vi "BuildPlotsOneGraph.vi"(0 "PlotCommand":string, 1 "Desired Legends":string[](array[string]), 2 "Error Bar Type":T1, 5 "Plotstyles":T3[](array[typedef]) {"LineType" min=1 max=6 step=1; "LineWidth" min=1 max=6 step=1; "PointSize" min=0 step=0.1}, 7 "PlotNamesNeed $$?":bool=TRUE, 9 "Plot Legends":string[](array[string]), 11 "PlotArray":cluster{dbl[], dbl[]}[](array[cluster]), 12 "Legend":string[](array[string]), 13 "Error Bar Cluster":T2[](array[typedef])) -> (4 "String out":string, 6 "Xspan":cluster{"Max":dbl, "Min":dbl}, 10 "Yspan":cluster{"Max":dbl, "Min":dbl})   [LabVIEW 2016]
uses:
  plotstyle.ctl
  Error_bars.ctl
  Error bar Type.ctl
  Results_plotter_Global.vi
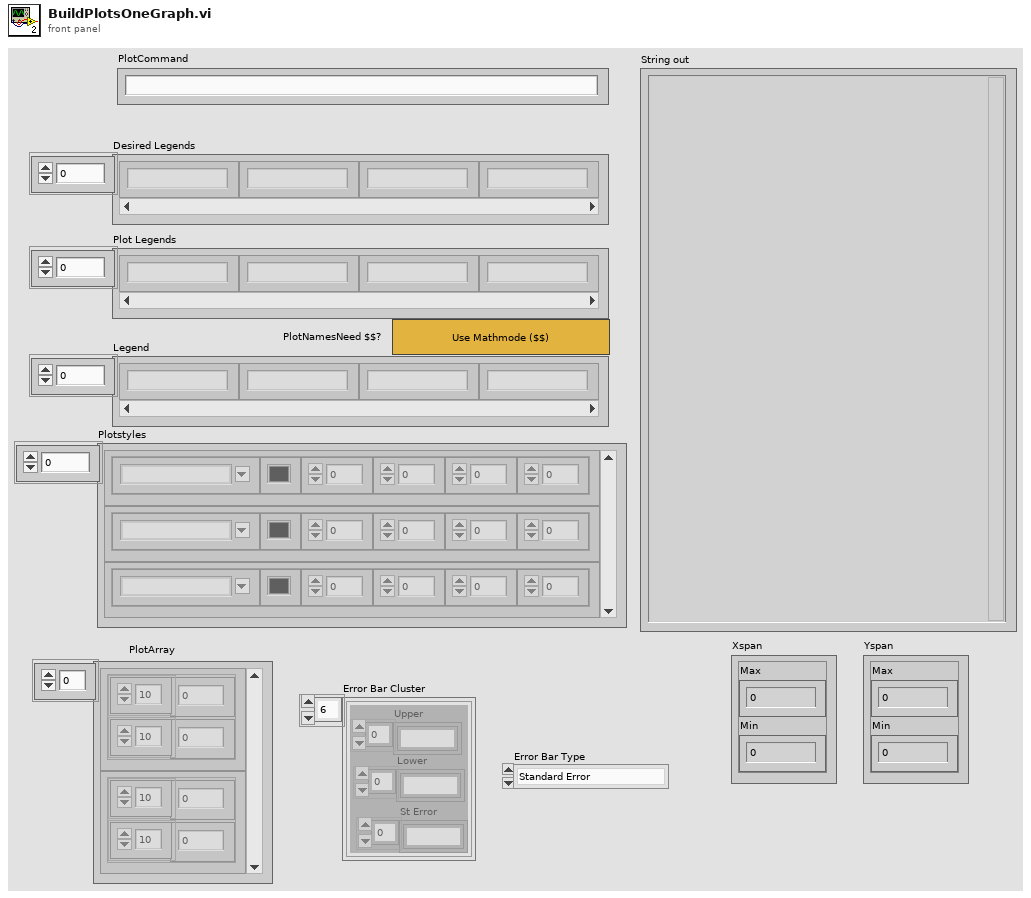
[diagram p1: front panel]
types:
  T1 = typedef "Error bar Type.ctl" = enum16{"Standard Error", "Separate upper and lower"}
  T2 = typedef "Error_bars.ctl" = cluster{"Upper":string[], "Lower":string[], "St Error":string[]}
  T3 = typedef "plotstyle.ctl" = cluster{"Style":string, "Color":u32, "PointType":i32, "PointSize":sgl, "LineWidth":sgl, "LineType":u8}
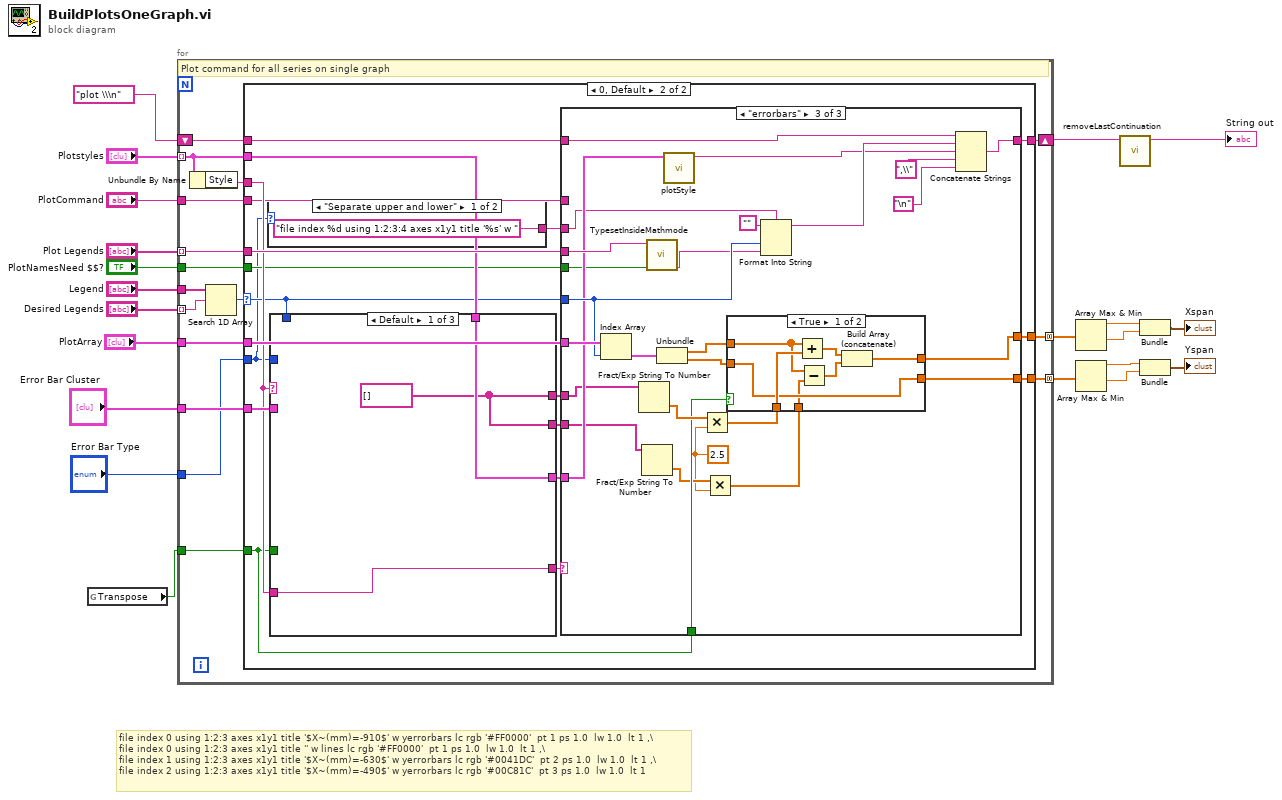
[diagram p0: block diagram]
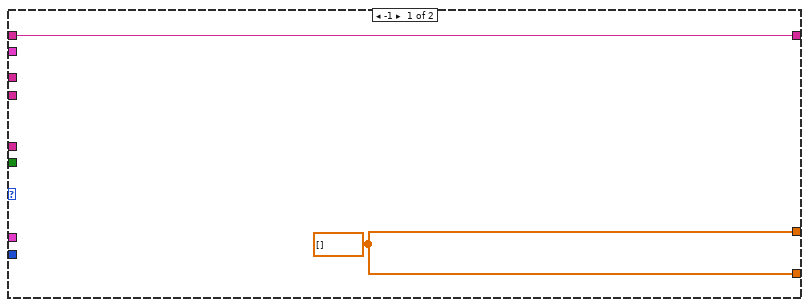
[diagram p2: hidden frame]
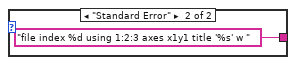
[diagram p3: hidden frame]
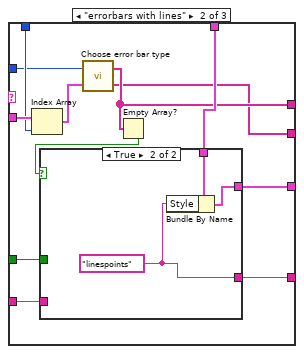
[diagram p4: hidden frame]
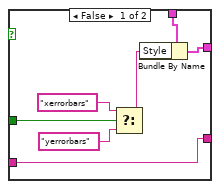
[diagram p5: hidden frame]
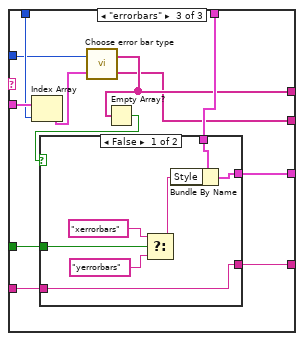
[diagram p6: hidden frame]
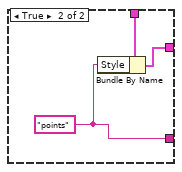
[diagram p7: hidden frame]
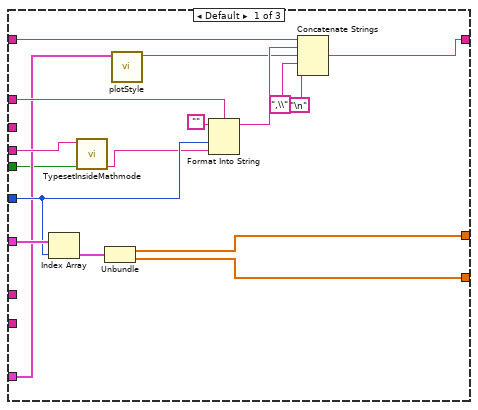
[diagram p8: hidden frame]
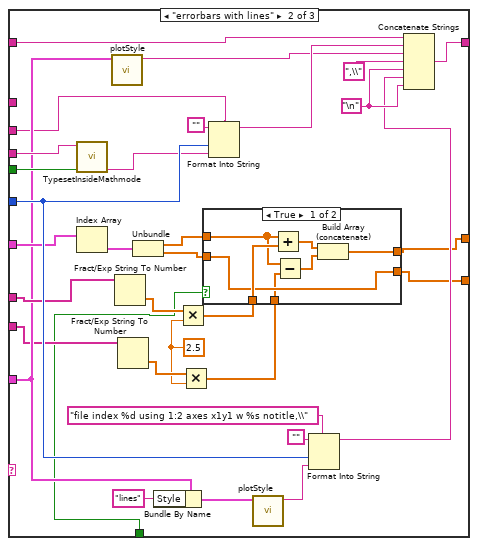
[diagram p9: hidden frame]
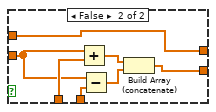
[diagram p10: hidden frame]
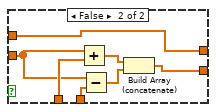
[diagram p11: hidden frame]
diagram:
  # "file index 0 using 1:2:3 axes x1y1 title '$X~(mm)=-910$' w yerrorbars lc rgb '#FF0000'  pt 1 ps 1.0  lw 1.0  lt 1 ,\\\nfile index 0 using 1:2:3 axes x1y1 title '' w lines lc rgb '#FF0000'  pt 1 ps 1.0  lw 1.0  lt 1 ,\\\nfile index 1 using 1:2:3 axes x1y1 title '$X~(mm)=-630$' w yerrorbars lc rgb '#0041DC'  pt 2 ps 1.0  lw 1.0  lt 1 ,\\\nfile index 2 using 1:2:3 axes x1y1 title '$X~(mm)=-490$' w yerrorbars lc rgb '#00C81C'  pt 3 ps 1.0  lw 1.0  lt 1"
  n1 = global read "Results_plotter_Global.vi" "Transpose"() -> (w3:bool)
  n2 = for {
    tunnel: "Plotstyles" -> [w27] mode=indexing
    tunnel: "Plot Legends" -> [w35] mode=indexing
    shift-right: [w36] -> w19
    shift-left: "plot \\\n" -> [w37]
    tunnel: "Desired Legends" -> [w33] mode=indexing
    tunnel: "Legend" -> [w34]
    tunnel: "PlotCommand" -> [w31]
    tunnel: "PlotArray" -> [w30]
    tunnel: [w29] -> w12 mode=concatenating
    tunnel: [w28] -> w11 mode=concatenating
    tunnel: "Error Bar Cluster" -> [w25]
    tunnel: w3 -> [w24]
    tunnel: "PlotNamesNeed $$?" -> [w23]
    tunnel: "Error Bar Type" -> [w22]
    # "Plot command for all series on single graph"
    n3 = Unbundle By Name(w27) -> ("Style"=w26:string)
    n4 = Search 1D Array(1D array=w34, element=w33) -> (index of element=w32:i32)  [unwired: 1 in]
    n5 = case shown="0, Default" w32 {
      selector: w32 -> [_ w47]
      tunnel: w27 -> [_ w51]
      tunnel: w37 -> [w39 w58]
      tunnel: [w39 w57] -> w36
      tunnel: w35 -> [_ w53]
      tunnel: w31 -> [_ w45]
      tunnel: w30 -> [_ w56]
      tunnel: [w38 w55] -> w29
      tunnel: [w38 w54] -> w28
      tunnel: w26 -> [_ w48]
      tunnel: w25 -> [_ w52]
      tunnel: w24 -> [_ w44]
      tunnel: w23 -> [_ w43]
      tunnel: w22 -> [_ w41]
      frame -1 {
        w38 = dbl[] []
      }
      frame 0, Default {
        n6 = case shown="\"Separate upper and lower\"" w41 {
          tunnel: ["file index %d using 1:2:3:4 axes x1y1 title '%s' w " ("format string") "file index %d using 1:2:3 axes x1y1 title '%s' w " ("format string")] -> w40
          frame "Separate upper and lower" {
          }
          frame "Standard Error" {
          }
        }
        n7 = case shown="Default" w48 {
          tunnel: w52 -> [_ w75 w97]
          tunnel: w51 -> [w63 w71 w93]
          tunnel: [w63 w70 w92] -> w50
          tunnel: [w62 w73 w95] -> w49
          tunnel: w44 -> [_ w72 w94]
          tunnel: w48 -> [w62 w69 w91]
          tunnel: w47 -> [_ w68 w90]
          tunnel: [w61 w65 w87] -> w46
          tunnel: w41 -> [_ w66 w88]
          tunnel: [w61 w64 w86] -> w42
          frame Default {
            w61 = string[] []
          }
          frame "errorbars with lines" {
            n8 = Index Array(array=w75, index=w68) -> (element=w67:T2)
            n9 = call "Choose error bar type.vi"("Error_bars"=w67, "Error Bar Type"=w66) -> ("Lower"=w64:string[], "Upper"=w65:string[])
            n10 = Empty Array?(array=w65) -> (empty?=w74:bool)
            n11 = case shown="True" w74 {
              tunnel: [w76 w83] -> w73
              tunnel: w72 -> [w80 _]
              tunnel: w71 -> [w79 w85]
              tunnel: [w78 w84] -> w70
              tunnel: w69 -> [w76 _]
              frame False {
                n12 = Select(t="xerrorbars", s=w80, f="yerrorbars") -> (s? t:f=w77:string)
                n13 = Bundle By Name(cluster=w79, "Style"=w77) -> (w78:T3)
              }
              frame True {
                w83 = "linespoints" ("Style")
                n14 = Bundle By Name(cluster=w85, "Style"=w83) -> (w84:T3)
              }
            }
          }
          frame "errorbars" {
            n15 = Index Array(array=w97, index=w90) -> (element=w89:T2)
            n16 = call "Choose error bar type.vi"("Error_bars"=w89, "Error Bar Type"=w88) -> ("Lower"=w86:string[], "Upper"=w87:string[])
            n17 = Empty Array?(array=w87) -> (empty?=w96:bool)
            n18 = case shown="False" w96 {
              tunnel: [w98 w105] -> w95
              tunnel: w94 -> [w102 _]
              tunnel: w93 -> [w101 w107]
              tunnel: [w100 w106] -> w92
              tunnel: w91 -> [w98 _]
              frame False {
                n19 = Select(t="xerrorbars", s=w102, f="yerrorbars") -> (s? t:f=w99:string)
                n20 = Bundle By Name(cluster=w101, "Style"=w99) -> (w100:T3)
              }
              frame True {
                w105 = "points" ("Style")
                n21 = Bundle By Name(cluster=w107, "Style"=w105) -> (w106:T3)
              }
            }
          }
        }
        n22 = case shown="\"errorbars\"" w49 {
          tunnel: w58 -> [w119 w153 w194]
          tunnel: [w110 w152 w193] -> w57
          tunnel: w45 -> [w118 _ _]
          tunnel: w56 -> [w117 w132 w192]
          tunnel: w47 -> [w116 w148 w189]
          tunnel: [w114 w127 w181] -> w55
          tunnel: [w113 w126 w180] -> w54
          tunnel: w53 -> [w112 w151 w190]
          tunnel: w50 -> [w111 w130 w187]
          tunnel: w46 -> [_ w131 w186]
          tunnel: w44 -> [_ w128 w184]
          tunnel: w43 -> [w109 w142 w178]
          tunnel: w42 -> [_ w129 w176]
          tunnel: w40 -> [_ w125 w172]
          frame Default {
            n23 = Index Array(array=w117, index=w116) -> (element=w115:cluster{dbl[], dbl[]})
            n24 = call "TypesetInsideMathmode.vi"("Needs $$?"=w109, "DirtyString"=w112) -> ("ChosenStringtype"=w108:string)  [unwired: 7 in, 2 out]
            n25 = Unbundle(w115) -> (w114:dbl[], w113:dbl[])
            n26 = call "plotStyle.vi"("plotSpec"=w111) -> ("String"=w121:string)  [unwired: 10 in]
            n27 = Format Into String(format string=w118, initial string="", w116, w108) -> (resulting string=w122:string)  [unwired: 1 in, 1 out]
            n28 = Concatenate Strings(w119, w122, w121, ",\\" ("string"), "\n") -> (w110:string)
          }
          frame "errorbars with lines" {
            w134 = 2.5
            w144 = "\n"
            n29 = call "TypesetInsideMathmode.vi"("Needs $$?"=w142, "DirtyString"=w151) -> ("ChosenStringtype"=w141:string)  [unwired: 7 in, 2 out]
            n30 = Index Array(array=w132) -> (element=w140:cluster{dbl[], dbl[]})  [unwired: 1 in]
            n31 = call "plotStyle.vi"("plotSpec"=w130) -> ("String"=w154:string)  [unwired: 10 in]
            n32 = Fract/Exp String To Number(string=w131) -> (number=w139:dbl[])  [unwired: 3 in, 1 out]
            n33 = Fract/Exp String To Number(string=w129) -> (number=w135:dbl[])  [unwired: 3 in, 1 out]
            n34 = Unbundle(w140) -> (w138:dbl[], w136:dbl[])
            n35 = Bundle By Name(cluster=w130, "Style"="lines") -> (w147:T3)
            n36 = Multiply(x=w139, y=w134) -> (x*y=w137:dbl[])
            n37 = Multiply(x=w135, y=w134) -> (x*y=w133:dbl[])
            n38 = case shown="True" w128 {
              tunnel: w138 -> [w161 w168]
              tunnel: w137 -> [w162 w169]
              tunnel: [w160 w168] -> w127
              tunnel: [w159 w166] -> w126
              tunnel: w136 -> [w159 w167]
              tunnel: w133 -> [w158 w165]
              frame True {
                n39 = Add(x=w161, y=w162) -> (x+y=w163:dbl[])
                n40 = Subtract(x=w161, y=w158) -> (x-y=w164:dbl[])
                n41 = Build Array (concatenate)(w163, w164) -> (w160:dbl[])
              }
              frame False {
                n42 = Add(x=w167, y=w169) -> (x+y=w170:dbl[])
                n43 = Subtract(x=w167, y=w165) -> (x-y=w171:dbl[])
                n44 = Build Array (concatenate)(w170, w171) -> (w166:dbl[])
              }
            }
            n45 = Format Into String(format string=w125, initial string="", w148, w141) -> (resulting string=w155:string)  [unwired: 1 in, 1 out]
            n46 = call "plotStyle.vi"("plotSpec"=w147) -> ("String"=w145:string)  [unwired: 10 in]
            n47 = Format Into String(format string="file index %d using 1:2 axes x1y1 w %s notitle,\\", initial string="", w148, w145) -> (resulting string=w143:string)  [unwired: 1 in, 1 out]
            n48 = Concatenate Strings(w153, w155, w154, ",\\" ("string"), w144, w143, w144) -> (w152:string)
          }
          frame "errorbars" {
            w174 = 2.5
            n49 = Index Array(array=w192, index=w189) -> (element=w191:cluster{dbl[], dbl[]})
            n50 = Fract/Exp String To Number(string=w186) -> (number=w185:dbl[])  [unwired: 3 in, 1 out]
            n51 = Fract/Exp String To Number(string=w176) -> (number=w175:dbl[])  [unwired: 3 in, 1 out]
            n52 = call "TypesetInsideMathmode.vi"("Needs $$?"=w178, "DirtyString"=w190) -> ("ChosenStringtype"=w177:string)  [unwired: 7 in, 2 out]
            n53 = Unbundle(w191) -> (w183:dbl[], w179:dbl[])
            n54 = call "plotStyle.vi"("plotSpec"=w187) -> ("String"=w195:string)  [unwired: 10 in]
            n55 = Multiply(x=w185, y=w174) -> (x*y=w182:dbl[])
            n56 = Multiply(x=w175, y=w174) -> (x*y=w173:dbl[])
            n57 = case shown="True" w184 {
              tunnel: w183 -> [w202 w209]
              tunnel: w182 -> [w203 w210]
              tunnel: [w201 w209] -> w181
              tunnel: [w200 w207] -> w180
              tunnel: w179 -> [w200 w208]
              tunnel: w173 -> [w199 w206]
              frame True {
                n58 = Add(x=w202, y=w203) -> (x+y=w204:dbl[])
                n59 = Subtract(x=w202, y=w199) -> (x-y=w205:dbl[])
                n60 = Build Array (concatenate)(w204, w205) -> (w201:dbl[])
              }
              frame False {
                n61 = Add(x=w208, y=w210) -> (x+y=w211:dbl[])
                n62 = Subtract(x=w208, y=w206) -> (x-y=w212:dbl[])
                n63 = Build Array (concatenate)(w211, w212) -> (w207:dbl[])
              }
            }
            n64 = Format Into String(format string=w172, initial string="", w189, w177) -> (resulting string=w196:string)  [unwired: 1 in, 1 out]
            n65 = Concatenate Strings(w194, w196, w195, ",\\" ("string"), "\n") -> (w193:string)
          }
        }
      }
    }
  }
  n66 = Array Max & Min(array=w12) -> (max value=w9:dbl, min value=w8:dbl)  [unwired: 2 out]
  n67 = Array Max & Min(array=w11) -> (max value=w7:dbl, min value=w6:dbl)  [unwired: 2 out]
  n68 = call "removeLastContinuation.vi"("String in"=w19) -> ("String out"=→"String out":string)  [unwired: 10 in]
  n69 = Bundle(w9, w8) -> (→"Xspan":cluster{dbl, dbl})  [unwired: 1 in]
  n70 = Bundle(w7, w6) -> (→"Yspan":cluster{dbl, dbl})  [unwired: 1 in]
